vi "InsertIntoPrepare.vi"(8 "error in (no error)":errorcluster, 9 "Items":string[](array[string]), 10 "Table Name":string, 11 "SQLite Connection in":refnum<class "Connection.lvclass">) -> (0 "error out":errorcluster, 2 "SQL Statement out":refnum<class "SQL Statement.lvclass">, 3 "SQLite Connection out":refnum<class "Connection.lvclass">)   [LabVIEW 2015, in "DBToolkit.lvlib"]
uses:
  DBToolkit.lvlib
  <vilib>/drjdpowell/SQLite Library/SQL Connection/Connection.lvclass
  <vilib>/drjdpowell/SQLite Library/SQL Statement/SQL Statement.lvclass
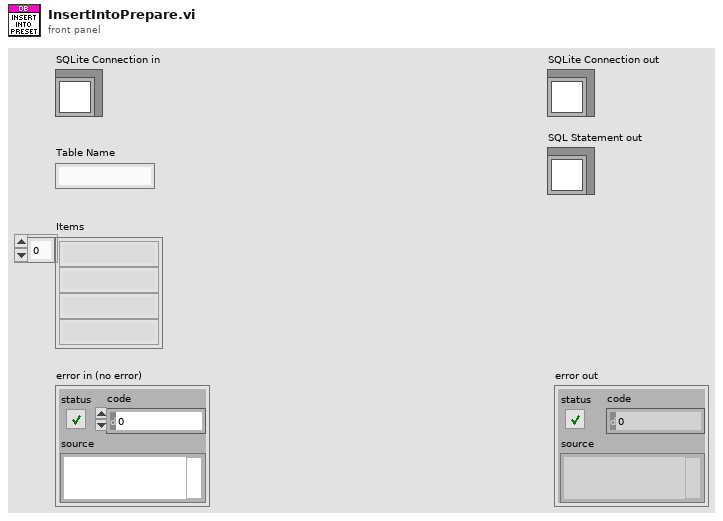
[diagram p1: front panel]
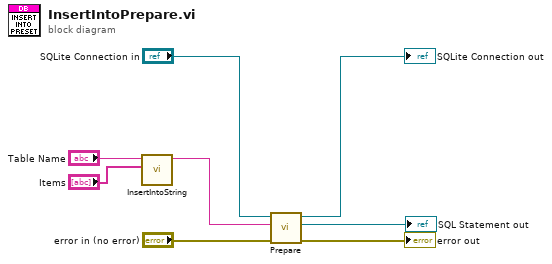
[diagram p0: block diagram]
diagram:
  n1 = call "InsertIntoString.vi"("Items"="Items", "Table Name"="Table Name") -> ("Insert Into String"=w5:string)  [unwired: 9 in]
  n2 = call <vilib>:"Prepare.vi"("error in (no error)"="error in (no error)", "SQL"=w5, "SQLite Connection in"="SQLite Connection in") -> ("error out"=→"error out":errorcluster, "SQL Statement out"=→"SQL Statement out":refnum<class "SQL Statement.lvclass">, "SQLite Connection out"=→"SQLite Connection out":refnum<class "Connection.lvclass">)  [unwired: 4 in, 2 out]
